vi "画图.vi"(7 "线段":cluster{i32, i32}[](array[cluster]), 8 "log":bool, 9 "Y轴":u16(ring) items=["Time", "Voltage", "Current"], 10 "X轴":u16(ring) items=["Time", "Voltage", "Current"], 11 "扫描数据":dbl[][](array[numeric])) -> (3 "XY图":picture)   [LabVIEW 2020]
uses:
  <vilib>/picture/cartesn2.llb/XY Plot Type.ctl
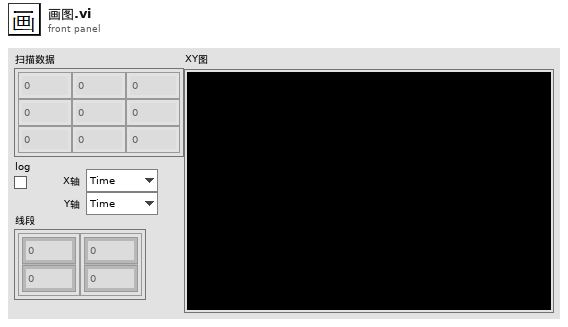
[diagram p1: front panel]
types:
  T1 = cluster{"line color":u32, "text color":u32, "tick length(3)":i16, "crossing axes":bool, "visible grid?":bool}
  T2 = cluster{"x minimum":dbl, "x maximum":dbl, "x log?":bool, "x precision":u8, "x format":enum8{"Decimal", "Scientific", "Engineering", "Binary", "Octal", "Hex"}, "y minimum":dbl, "y maximum":dbl, "y log?":bool, "y precision":u8, "y format":enum8{"Decimal", "Scientific", "Engineering", "Binary", "Octal", "Hex"}}
  T3 = typedef "XY Plot Type.ctl" = enum16{"points", "squares", "circles", "connected points", "connected squares", "connected circles", "comb plot", "sized scatter plot", "sized-colored scatter plot", "min-max lines"}
  T4 = cluster{"plot color":u32, "XY plot type":T3, "baseline":dbl}[]
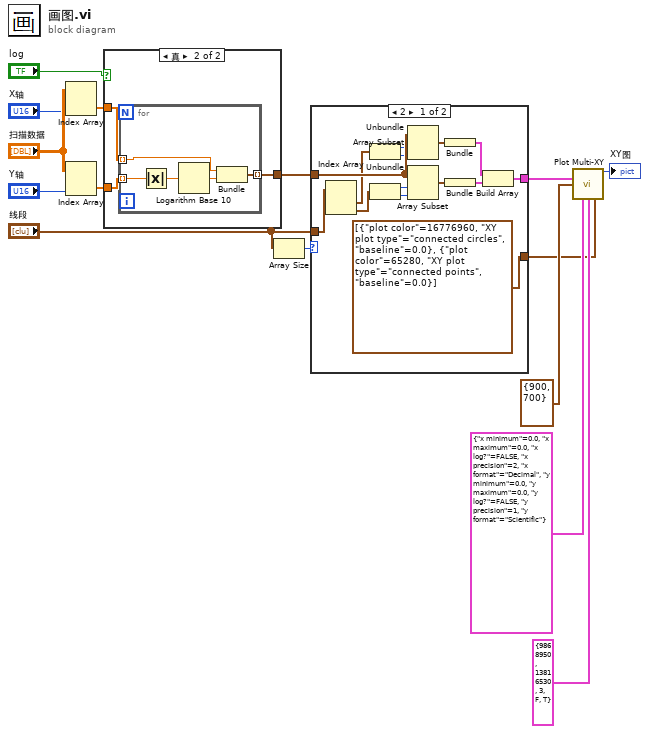
[diagram p0: block diagram]
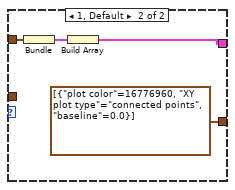
[diagram p2: hidden frame]
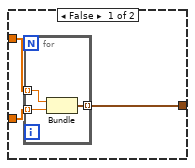
[diagram p3: hidden frame]
diagram:
  n1 = Index Array(array="扫描数据", index (col)="X轴") -> (element=w14:dbl[])  [unwired: 1 in]
  n2 = Index Array(array="扫描数据", index (col)="Y轴") -> (element=w15:dbl[])  [unwired: 1 in]
  n3 = case shown="真" "log" {
    tunnel: w15 -> [w18 w23]
    tunnel: w14 -> [w17 w24]
    tunnel: [w16 w22] -> w13
    frame False {
      n4 = for {
        tunnel: [w21] -> w16 mode=indexing
        tunnel: w17 -> [w20] mode=indexing
        tunnel: w18 -> [w19] mode=indexing
        n5 = Bundle(w20, w19) -> (w21:cluster{dbl, dbl})  [unwired: 1 in]
      }
    }
    frame True {
      n6 = for {
        tunnel: w24 -> [w29] mode=indexing
        tunnel: w23 -> [w26] mode=indexing
        tunnel: [w28] -> w22 mode=indexing
        n7 = Absolute Value(x=w26) -> (abs(x)=w27:dbl)
        n8 = Logarithm Base 10(1:w27) -> (0:w25:dbl)
        n9 = Bundle(w29, w25) -> (w28:cluster{dbl, dbl})  [unwired: 1 in]
      }
    }
  }
  n10 = Array Size(array="线段") -> (size(s)=w3:i32)
  n11 = case shown="2" w3 {
    tunnel: w13 -> [w43 w47]
    tunnel: [w38 w45] -> w12
    tunnel: "线段" -> [w37 _]
    tunnel: [T4 [{"plot color"=16776960, "XY plot type"=enum."connected circles", "baseline"=0.0}, {"plot color"=65280, "XY plot type"=enum."connected points", "baseline"=0.0}] ("XY plot cosmetics") T4 [{"plot color"=16776960, "XY plot type"=enum."connected points", "baseline"=0.0}] ("XY plot cosmetics")] -> w2
    frame 2 {
      n12 = Index Array(array=w37) -> (element #1=w36:cluster{i32, i32}, element #2=w33:cluster{i32, i32})  [unwired: 2 in]
      n13 = Unbundle(w36) -> (w35:i32, w34:i32)
      n14 = Unbundle(w33) -> (w32:i32, w31:i32)
      n15 = Array Subset(array=w43, index=w35, length=w34) -> (w42:cluster{dbl, dbl}[])
      n16 = Array Subset(array=w43, index=w32, length=w31) -> (w41:cluster{dbl, dbl}[])
      n17 = Bundle(w42) -> (w40:cluster{cluster{dbl, dbl}[]})  [unwired: 1 in]
      n18 = Bundle(w41) -> (w39:cluster{cluster{dbl, dbl}[]})  [unwired: 1 in]
      n19 = Build Array(w40, w39) -> (w38:cluster{cluster{dbl, dbl}[]}[])
    }
    frame 1, Default {
      n20 = Bundle(w47) -> (w46:cluster{cluster{dbl, dbl}[]})  [unwired: 1 in]
      n21 = Build Array(w46) -> (w45:cluster{cluster{dbl, dbl}[]}[])
    }
  }
  n22 = call <vilib>:"Plot Multi-XY.vi"("data"=w12, "dimensions (w,h)"=cluster{"width":i16, "height":i16} {"width"=900, "height"=700}, "cartesian axis attributes"=T2 {"x minimum"=0.0, "x maximum"=0.0, "x log?"=FALSE, "x precision"=2, "x format"=enum."Decimal", "y minimum"=0.0, "y maximum"=0.0, "y log?"=FALSE, "y precision"=1, "y format"=enum."Scientific"}, "cartesian grid cosmetics"=T1 {"line color"=9868950, "text color"=13816530, "tick length(3)"=3, "crossing axes"=FALSE, "visible grid?"=TRUE}, "XY plot cosmetics"=w2) -> ("new picture"=→"XY图":picture)  [unwired: 10 in]
